vi "ADFX_Do_Load.vi"(8 "error in (no error)":errorcluster, 11 "Data in":T1) -> (0 "error out":errorcluster, 3 "Data out":T1)   [LabVIEW 2015]
doc: "Reads and sets control data from save file."
uses:
  controls/AFXP Data.ctl
  controls/AFCP Setup.ctl
  <vilib>/Utility/sysdir.llb/System Directory Type.ctl
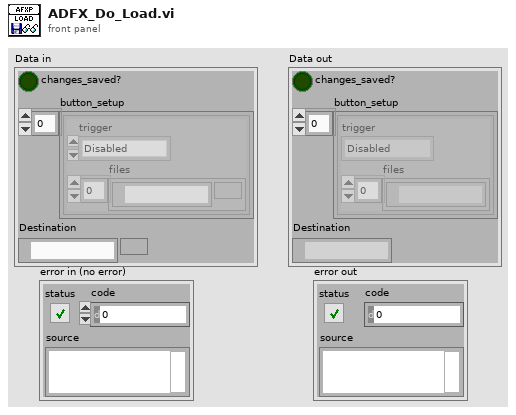
[diagram p1: front panel]
types:
  T1 = typedef "AFXP Data.ctl" = cluster{"changes_saved?":bool, "button_setup":T2[], "Destination":path}
  T2 = typedef "AFCP Setup.ctl" = cluster{"trigger":enum16{"Basic", "Hold-Loop", "Latch-Loop", "Next", "Random", "Disabled"}, "files":path[]}
  T3 = typedef "System Directory Type.ctl" = i32
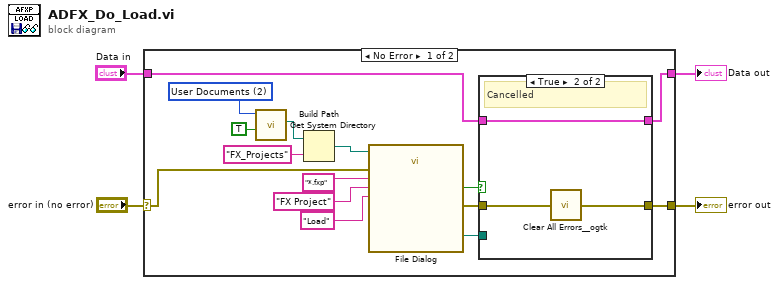
[diagram p0: block diagram]
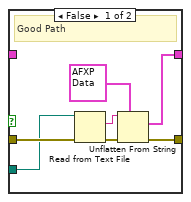
[diagram p2: hidden frame]
diagram:
  n1 = case shown="No Error" "error in (no error)" {
    selector: "error in (no error)" -> [w8 w31]
    tunnel: "Data in" -> [w19 w30]
    tunnel: [w11 w31] -> w3
    tunnel: [w9 w30] -> w2
    frame No Error {
      w6 = T3 2 items=["User Home"=0, "User Desktop"=1, "User Documents"=2, "User Application Data"=3, "User Preferences"=4, "User Temporary"=5, "Public Documents"=6, "Public Application Data"=7, "Public Preferences"=8, "Public Cache"=13, "System Core Libraries"=9, "System Installed Libraries"=10, "Application Files"=11, "Boot Volume Root"=12] ("system directory type")
      n2 = call <vilib>:"Get System Directory.vi"("create directory if not found? (F)"=TRUE, "system directory type"=w6) -> ("system directory"=w5:path)  [unwired: 9 in]
      n3 = Build Path(base path=w5, name or relative path="FX_Projects") -> (appended path=w18:path)
      n4 = call "File Dialog"("start path"=w18, "button label"="Load", "error in"=w8, "pattern (all files)"="*.fxp", "pattern label"="FX Project") -> ("selected path"=w12:path, "cancelled"=w17:bool, "error out"=w10:errorcluster)  [unwired: 7 in, 1 out]
      n5 = case shown="True" w17 {
        tunnel: w10 -> [w26 w29]
        tunnel: [w23 w27] -> w11
        tunnel: w12 -> [w25 _]
        tunnel: w19 -> [_ w28]
        tunnel: [w20 w28] -> w9
        frame False {
          # "Good Path"
          n6 = Read from Text File(file (use dialog)=w25, error in=w26) -> (text=w22:string, error out=w24:errorcluster)  [unwired: 2 in, 2 out]
          n7 = Unflatten From String(type=T1 {"changes_saved?"=TRUE, "button_setup"=[{"trigger"=enum."Basic", "files"=[]}, {"trigger"=enum."Basic", "files"=[]}, {"trigger"=enum."Basic", "files"=[]}, {"trigger"=enum."Basic", "files"=[]}, {"trigger"=enum."Basic", "files"=[]}, {"trigger"=enum."Basic", "files"=[]}, {"trigger"=enum."Basic", "files"=[]}, {"trigger"=enum."Basic", "files"=[]}, {"trigger"=enum."Basic", "files"=[]}, {"trigger"=enum."Basic", "files"=[]}, {"trigger"=enum."Basic", "files"=[]}, {"trigger"=enum."Basic", "files"=[]}, {"trigger"=enum."Basic", "files"=[]}], "Destination"=path ""} ("Data"), binary string=w22, error in (no error)=w24) -> (value=w20:T1, error out=w23:errorcluster)  [unwired: 2 in, 1 out]
        }
        frame True {
          # "Cancelled"
          n8 = call <userlib>:"Clear All Errors__ogtk.vi"("Error In"=w29) -> ("Error Out"=w27:errorcluster)  [unwired: 3 in]
        }
      }
    }
    frame Error {
    }
  }
  "error out" <- w3
  "Data out" <- w2
